vi "PmacCommAppend.vi"(0 "Response String":string, 1 "Command String":string) -> ()   [LabVIEW 2020]
doc: "Copy Command String and Response String to the last communication items in PmacCommGlobal. If Logging Enabled is TRUE they are also appended to the Communication Log."
uses:
  PmacCommGlobal.vi
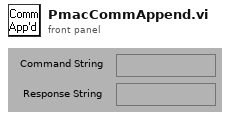
[diagram p1: front panel]
types:
  T1 = cluster{"Command String":string, "Response String":string, "Communication Log String":string, "Num Commands i32":i32, "Buffer Log Bool (F)":bool}
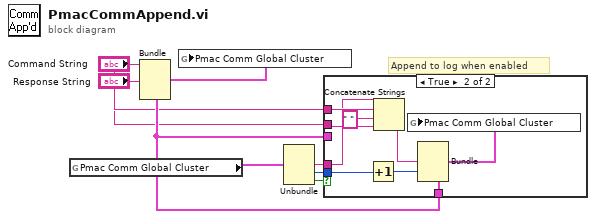
[diagram p0: block diagram]
diagram:
  # "Append to log when enabled"
  n1 = global read "PmacCommGlobal.vi" "Pmac Comm Global Cluster"() -> (w7:T1)
  n2 = Bundle(cluster=w7, "Command String"="Command String", "Response String"="Response String") -> (w3:T1)  [unwired: 3 out]
  n3 = global write "PmacCommGlobal.vi" "Pmac Comm Global Cluster"(w3) -> ()
  n4 = Unbundle(w7) -> ("Communication Log String"=w2:string, "Num Commands i32"=w1:i32, "Buffer Log Bool (F)"=w6:bool)  [unwired: 2 out]
  n5 = case shown="True" w6 {
    tunnel: w7 -> [_ _]
    tunnel: w2 -> [_ w12]
    tunnel: w1 -> [_ w16]
    tunnel: "Response String" -> [_ w14]
    tunnel: "Command String" -> [_ w13]
    tunnel: w7 -> [_ w10]
    frame False {
    }
    frame True {
      n6 = Increment(x=w16) -> (x+1=w9:i32)
      n7 = Concatenate Strings(w12, w13, " ", w14) -> (w8:string)
      n8 = Bundle(cluster=w10, "Communication Log String"=w8, "Num Commands i32"=w9) -> (w11:T1)  [unwired: 3 out]
      n9 = global write "PmacCommGlobal.vi" "Pmac Comm Global Cluster"(w11) -> ()
    }
  }
